vi "MB Ethernet Call Wait on Query.vi"(9 "Data Reference":T1, 10 "Timeout":i32=5000, 11 "Connection ID":refnum<k5>) -> ()   [LabVIEW 2019, in "NI_modbus_upd.lvlib"]
uses:
  NI_modbus_upd.lvlib
panel:
  # "VI Name: MB Ethernet Call Wait on Query.vi\nPurpose: Dynamically calls MB Ethernet Wait on Query.vi"
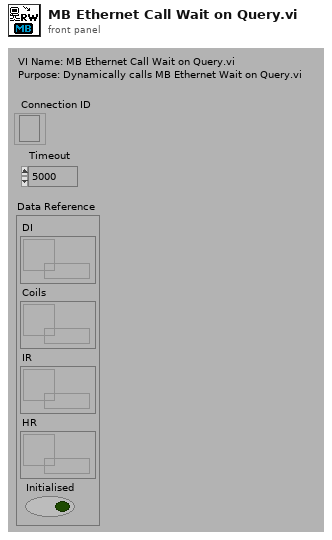
[diagram p1: front panel]
types:
  T1 = cluster{"DI":refnum<data-value>, "Coils":refnum<data-value>, "IR":refnum<data-value>, "HR":refnum<data-value>, "Initialised":bool}
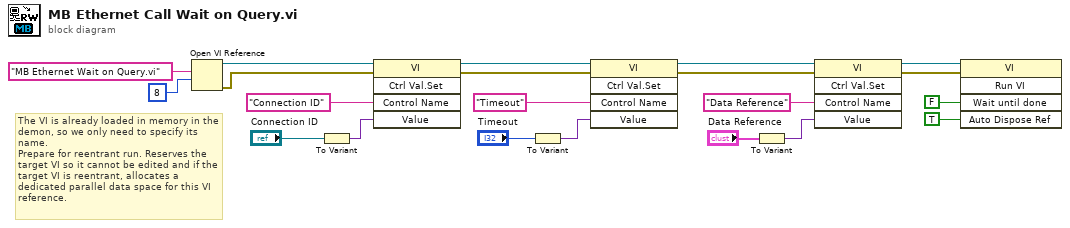
[diagram p0: block diagram]
diagram:
  # "The VI is already loaded in memory in the demon, so we only need to specify its name.\nPrepare for reentrant run. Reserves the target VI so it cannot be edited and if the target VI is reentrant, allocates a dedicated parallel data space for this VI reference."
  n1 = Open VI Reference(vi path="MB Ethernet Wait on Query.vi", options=8) -> (vi reference=w11:refnum<vi>, error out=w8:errorcluster)  [unwired: 4 in]
  n2 = To Variant(anything="Connection ID") -> (Variant=w19:variant)
  n3 = invoke class="VI" method="Ctrl Val.Set"(reference=w11, error in=w8, "Control Name"="Connection ID", "Value"=w19) -> (reference out=w10:refnum<vi>, error out=w9:errorcluster)  [unwired: 1 in, 3 out]
  n4 = To Variant(anything="Timeout") -> (Variant=w15:variant)
  n5 = invoke class="VI" method="Ctrl Val.Set"(reference=w10, error in=w9, "Control Name"="Timeout", "Value"=w15) -> (reference out=w5:refnum<vi>, error out=w4:errorcluster)  [unwired: 1 in, 3 out]
  n6 = To Variant(anything="Data Reference") -> (Variant=w6:variant)
  n7 = invoke class="VI" method="Ctrl Val.Set"(reference=w5, error in=w4, "Control Name"="Data Reference", "Value"=w6) -> (reference out=w3:refnum<vi>, error out=w2:errorcluster)  [unwired: 1 in, 3 out]
  n8 = invoke class="VI" method="Run VI"(reference=w3, error in=w2, "Wait until done"=FALSE, "Auto Dispose Ref"=TRUE) -> ()  [unwired: 1 in, 5 out]
